vi "ALLOW DRIVE.vi"(8 "error in (no error)":errorcluster, 10 "Cluster in":T3, 11 "FPGA Interface":T1) -> ()   [LabVIEW 2015]
uses:
  PC/QMH Fundamentals - Message Cluster.ctl
  <vilib>/RioEmbeddedCAN/RioEmbeddedCAN.llb/CANFrameControl.ctl
  fpga-type-def.ctl
  GLOBAL on RT.vi
  <vilib>/Utility/error.llb/Error Cluster From Error Code.vi
  <vilib>/rvi/errors/niLvFpgaAdjustHostInterfaceError.vi
  <vilib>/rvi/interface/nirviReadWriteControl/nirviReadWriteControl.xnode
  FPGA Bitfiles/Raptorv2_FPGATarget_FPGAMain_QFI8efjbaF8.lvbitx
  FPGA/Main FPGA.vi
  NiFpgaLv.dll
  <vilib>/Utility/Variable/NI_VariableUtilities.lvlib
panel:
  in  "reset stop manual":bool
  out "E-STOP ACTIVE":bool
  out "E-STOP Button":bool
  out "RESET E-STOP Button":bool
  in  "po jakim czasie załączyć":u64=1000
  in  "całkowity okres":u64=2000
  in  "zolta Lapmka":bool
  in  "stop manual":bool
  in  "zero v":T2[](array[typedef])=[{"identifier"=1, "extended?"=FALSE, "type"=0, "payload"=[1, 0, 0, 0, 0, 0, 0]}, {"identifier"=2, "extended?"=FALSE, "type"=0, "payload"=[1, 0, 0, 0, 0, 0, 0]}] {"type" items=["CAN Data", "CAN Remote"]; "identifier" format="%.0x"}
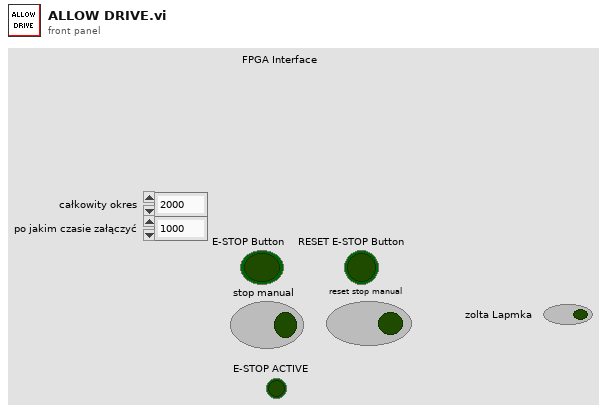
[diagram p1: front panel]
types:
  T1 = typedef "fpga-type-def.ctl" = refnum<k20>
  T2 = typedef "CANFrameControl.ctl" = cluster{"identifier":u32, "extended?":bool, "type":u8, "payload":u8[]}
  T3 = cluster{"DRIVE":refnum<queue>, "KONFIG,PROBE,ARM":refnum<queue>, "ERROR Q":errorcluster, "SEND DATA":refnum<queue>, "TIMEOUT":refnum<queue>, "GIMBALE":refnum<queue>, "SAFETY":refnum<queue>}
  T4 = typedef "QMH Fundamentals - Message Cluster.ctl" = cluster{"Message":string, "Message Data":variant}
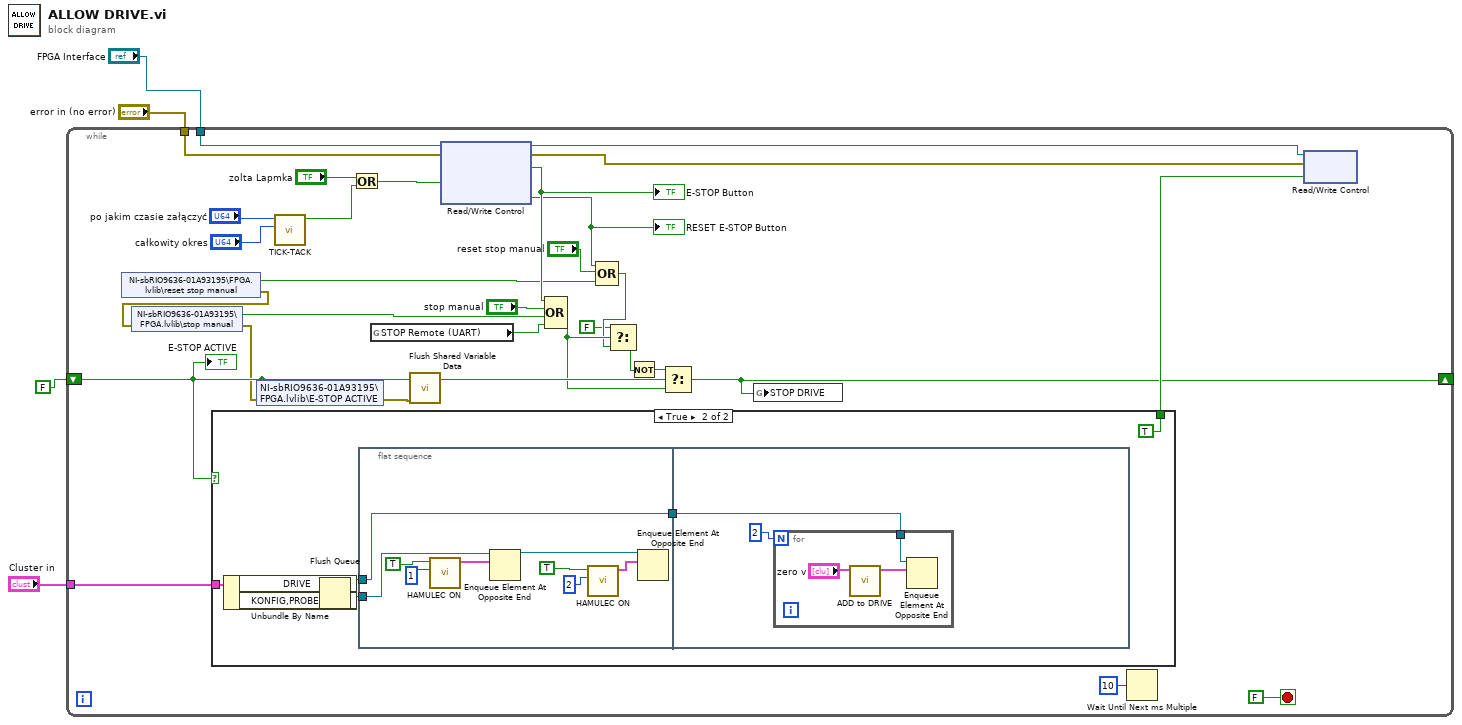
[diagram p0: block diagram]
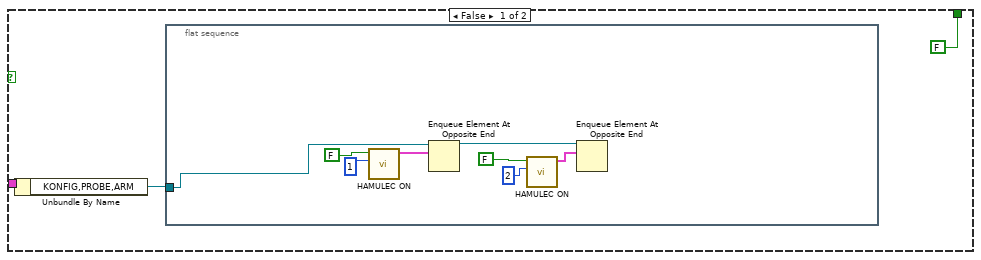
[diagram p2: hidden frame]
diagram:
  n1 = while {
    tunnel: "FPGA Interface" -> [w34]
    tunnel: "error in (no error)" -> [w33]
    tunnel: "Cluster in" -> [w31]
    shift-right: [w19] -> _
    shift-left: FALSE -> [w24]
    stop <- FALSE stop-if-true
    n2 = shared-variable "NI-sbRIO9636-01A93195\\FPGA.lvlib\\reset stop manual"() -> (w14:bool, error out=w15:errorcluster)  [unwired: 1 in]
    n3 = shared-variable "NI-sbRIO9636-01A93195\\FPGA.lvlib\\stop manual"(error in=w15) -> (w13:bool, error out=w8:errorcluster)
    n4 = case shown="True" w24 {
      tunnel: w31 -> [w37 w50]
      tunnel: [FALSE TRUE] -> w20
      frame False {
        n5 = Unbundle By Name(w37) -> ("KONFIG,PROBE,ARM"=w36:refnum<queue>)
        n6 = flat-sequence {
          tunnel: w36 -> [w43]
          frame #0 {
            n7 = call "HAMULEC ON.vi"("identifier"=u32 1 ("lewa/prawa"), "Hamulec ON"=FALSE) -> ("Message Cluster"=w42:T4)  [unwired: 9 in]
            n8 = Enqueue Element At Opposite End(queue=w43, element=w42) -> (queue out=w39:refnum<queue>)  [unwired: 2 in, 2 out]
            n9 = call "HAMULEC ON.vi"("identifier"=u32 2 ("lewa/prawa"), "Hamulec ON"=FALSE) -> ("Message Cluster"=w38:T4)  [unwired: 9 in]
            n10 = Enqueue Element At Opposite End(queue=w39, element=w38) -> ()  [unwired: 2 in, 3 out]
          }
        }
      }
      frame True {
        n11 = Unbundle By Name(w50) -> ("DRIVE"=w49:refnum<queue>, "KONFIG,PROBE,ARM"=w48:refnum<queue>)
        n12 = Flush Queue(queue=w49) -> ()  [unwired: 1 in, 3 out]
        n13 = flat-sequence {
          tunnel: w48 -> [w52]
          tunnel: w49 -> [w51]
          tunnel: [w51] -> w47
          tunnel: w47 -> [w61]
          frame #0 {
            n14 = call "HAMULEC ON.vi"("identifier"=u32 1 ("lewa/prawa"), "Hamulec ON"=TRUE) -> ("Message Cluster"=w55:T4)  [unwired: 9 in]
            n15 = Enqueue Element At Opposite End(queue=w52, element=w55) -> (queue out=w58:refnum<queue>)  [unwired: 2 in, 2 out]
            n16 = call "HAMULEC ON.vi"("identifier"=u32 2 ("lewa/prawa"), "Hamulec ON"=TRUE) -> ("Message Cluster"=w59:T4)  [unwired: 9 in]
            n17 = Enqueue Element At Opposite End(queue=w58, element=w59) -> ()  [unwired: 2 in, 3 out]
          }
          frame #1 {
            n18 = for {
              N: 2 -> [_]
              tunnel: w61 -> [w62]
              n19 = call "ADD to DRIVE.vi"("zero v"="zero v") -> ("Message Cluster"=w63:T4)  [unwired: 10 in]
              n20 = Enqueue Element At Opposite End(queue=w62, element=w63) -> ()  [unwired: 2 in, 3 out]
            }
          }
        }
      }
    }
    n21 = shared-variable "NI-sbRIO9636-01A93195\\FPGA.lvlib\\E-STOP ACTIVE"(w24, error in=w8) -> (error out=w6:errorcluster)
    n22 = call "TICK-TACK.vi"("calkowity okres"="całkowity okres", "czas załaczenia"="po jakim czasie załączyć") -> ("Timeout"=w26:bool)  [unwired: 9 in]
    n23 = Or(x="zolta Lapmka", y=w26) -> (x .or. y?=w27:bool)
    n24 = global read "GLOBAL on RT.vi" "STOP Remote (UART)"() -> (w5:bool)
    n25 = call <vilib>:"Flush Shared Variable Data.vi"("error in (no error)"=w6) -> ()  [unwired: 10 in, 1 out]
    n26 = xnode "Read/Write Control"("FPGA VI Reference In"=w34, "error in"=w33, "DIO21"=w27) -> ("FPGA VI Reference Out"=w22:T1, "error out"=w21:errorcluster, "STOP ??"=w17:bool, "Reset stop 25"=w16:bool)
    "RESET E-STOP Button" <- w16
    "E-STOP Button" <- w17
    n27 = Compound Arithmetic op=OR(w17, "stop manual", w13, w5) -> (w12:bool)
    n28 = Compound Arithmetic op=OR(w16, "reset stop manual", w14) -> (w10:bool)
    n29 = Select(t=FALSE, s=w12, f=w10) -> (s? t:f=w11:bool)
    n30 = Not(x=w11) -> (.not. x?=w23:bool)
    n31 = Select(t=w23, s=w24, f=w12) -> (s? t:f=w19:bool)
    n32 = global write "GLOBAL on RT.vi" "STOP DRIVE"(w19) -> ()
    n33 = Wait Until Next ms Multiple(millisecond multiple=u32 10) -> ()  [unwired: 1 out]
    n34 = xnode "Read/Write Control"("FPGA VI Reference In"=w22, "error in"=w21, "DIO22"=w20) -> ()  [unwired: 2 out]
    "E-STOP ACTIVE" <- w24
  }
